vi "UnifyIterator.vi"(7 "Actor in":refnum<class "Actor.lvclass">, 9 "Unify in":T1, 10 "Actors":refnum<class "Actor.lvclass">[](array[class])) -> (1 "Unify out":T1, 5 "Actor out":refnum<class "Actor.lvclass">)   [LabVIEW 2020, in "jettl.lvlib"]
uses:
  jettl.lvlib
  Message/Message.lvclass
  Actor/Actor.lvclass
  MessageSet.ctl
  Messages.ctl
  Unify.ctl
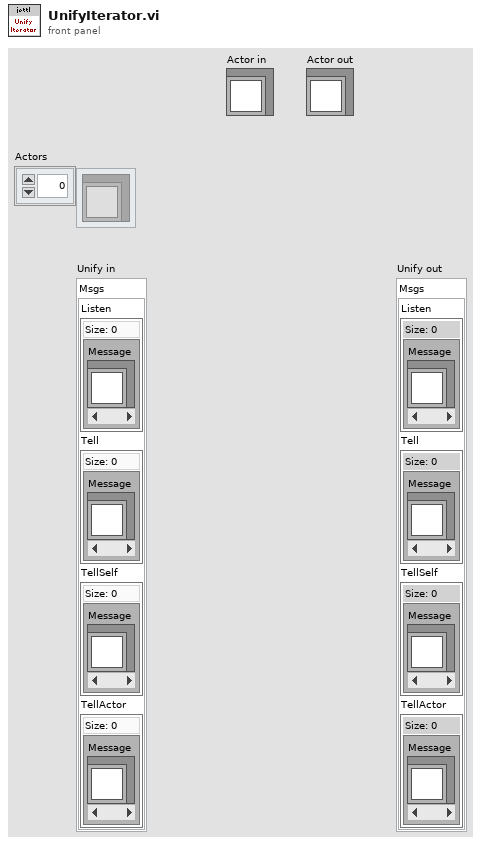
[diagram p1: front panel]
types:
  T1 = typedef "jettl.lvlib/Unify.ctl" = cluster{"Msgs":T2}
  T2 = typedef "jettl.lvlib/Messages.ctl" = cluster{"Listen":T3, "Tell":T3, "TellSelf":T3, "TellActor":T3}
  T3 = typedef "jettl.lvlib/MessageSet.ctl" = set{refnum<class "Message.lvclass">}
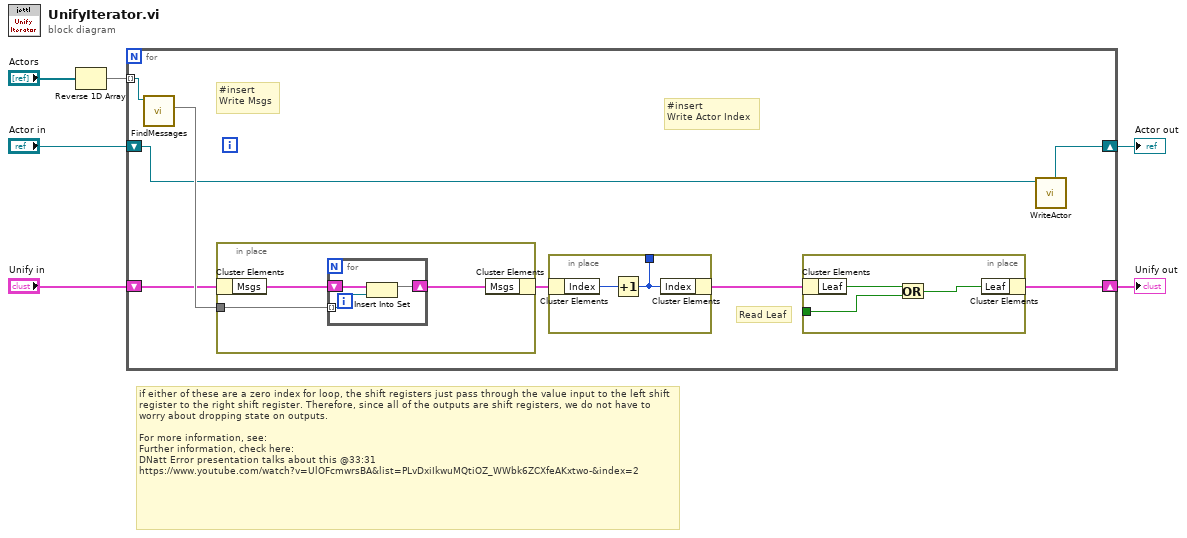
[diagram p0: block diagram]
diagram:
  # "if either of these are a zero index for loop, the shift registers just pass through the value input to the left shift register to the right shift register. Therefore, since all of the outputs are shift registers, we do not have to worry about dropping state on outputs.\n\nFor more information, see:\nFurther information, check here:\nDNatt Error presentation talks about this @33:31\nhttps://www.youtube.com/watch?v=UlOFcmwrsBA&list=PLvDxiIkwuMQtiOZ_WWbk6ZCXfeAKxtwo-&index=2"
  n1 = Reverse 1D Array(array="Actors") -> (reversed array=w6:refnum<class "Actor.lvclass">[])
  n2 = for {
    tunnel: w6 -> [w15] mode=indexing
    shift-right: [w9] -> w5
    shift-left: "Actor in" -> [w7]
    shift-right: [w16] -> w1
    shift-left: "Unify in" -> [w10]
    # "#insert\nWrite Actor Index"
    # "#insert\nWrite Msgs"
    # "Read Leaf"
    n3 = call-dynamic "FindMessages.vi"(11:w15) -> (2:w17)  [unwired: 9 in, 1 out]
    n4 = in-place {
      in-place-border: w17 -> [w25]
      n5 = in-place-cluster #1(w10) -> ("Msgs"=w24:T2)
      n6 = for {
        shift-right: [w27] -> w23
        shift-left: w24 -> [w28]
        tunnel: w25 -> [w26] mode=indexing
        n7 = Insert Into Set(10:w26, 11:w28) -> (3:w27:set{refnum<class "Message.lvclass">})  [unwired: 1 out]
      }
      n8 = in-place-cluster #1("Msgs"=w23) -> (w13:T1)
    }
    n9 = in-place {
      in-place-border: [w21] -> w11
      n10 = in-place-cluster #2(w13) -> ("Index"=w22:i32)
      n11 = Increment(x=w22) -> (x+1=w21:i32)
      n12 = in-place-cluster #2("Index"=w21) -> (w12:T1)
    }
    n13 = in-place {
      in-place-border: [w18] -> w14
      n14 = in-place-cluster #3(w12) -> ("Leaf"=w20:bool)
      n15 = Or(x=w20, y=w18) -> (x .or. y?=w19:bool)
      n16 = in-place-cluster #3("Leaf"=w19) -> (w16:T1)
    }
    n17 = call-dynamic "WriteActor.vi"("Actor"=w7) -> ("Actor out"=w9:refnum<class "Actor.lvclass">, "Actor in"=w8:refnum<class "Actor.lvclass">)  [unwired: 9 in]
  }
  "Actor out" <- w5
  "Unify out" <- w1
